vi "Serial connection test.vi"() -> ()   [LabVIEW 2024]
uses:
  664af4c5-80d0-43d0-860f-6e657b5a4ca0.vi
  <vilib>/regexp/Match Regular Expression.xnode
panel:
  out "error out":errorcluster
  out "find list":string[](array[string])
  in  "error in (no error)":errorcluster
  out "Device describtion":string[](array[string])
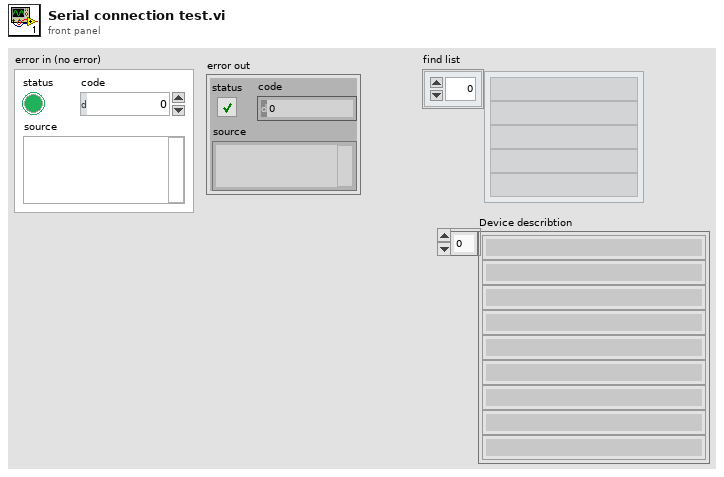
[diagram p1: front panel]
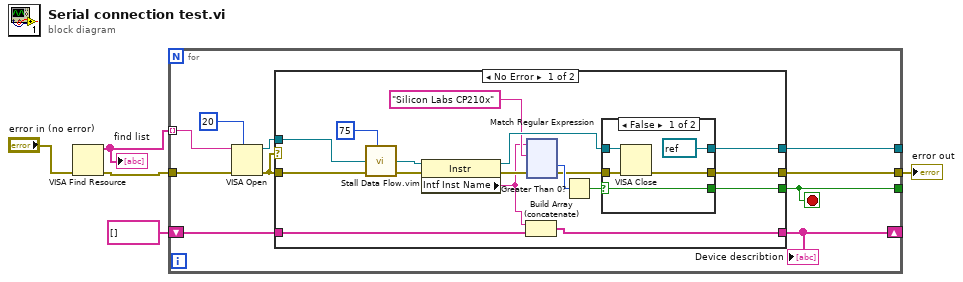
[diagram p0: block diagram]
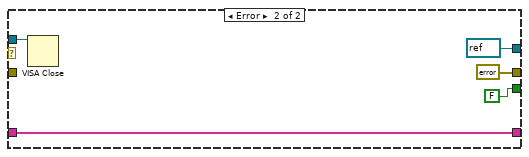
[diagram p3: hidden frame]
diagram:
  n1 = VISA Find Resource(8:"error in (no error)") -> (0:w4:errorcluster, 3:w5:string[])  [unwired: 2 in, 1 out]
  "find list" <- w5
  n2 = for {
    tunnel: w5 -> [w15] mode=indexing
    tunnel: w4 -> [w14]
    tunnel: [w11] -> w2
    tunnel: [w10] -> _
    tunnel: [w12] -> _
    shift-right: [w7] -> _
    shift-left: string[] [] -> [w6]
    stop <- w10 stop-if-true
    n3 = VISA Open(timeout (0)=u32 20 ("VISA Open timeout (0)"), error in (no error)=w14, VISA resource name=w15) -> (VISA resource name=w9:refnum<visa-resource-name>, error out=w13:errorcluster)  [unwired: 2 in]
    n4 = case shown="No Error" w13 {
      tunnel: w9 -> [w21 w159]
      tunnel: w13 -> [w31 _]
      tunnel: [w28 refnum<visa-resource-name> refnum ("Port")] -> w12
      tunnel: [w27 FALSE] -> w10
      tunnel: [w26 errorcluster {"status"=FALSE, "code"=0, "source"=""} ("error out")] -> w11
      tunnel: [w17 w157] -> w7
      tunnel: w6 -> [w16 w157]
      frame No Error {
        n5 = call "Stall Data Flow.vim"("value in"=w21, "milliseconds to wait"=u32 75) -> ("value out"=w20:refnum<visa-resource-name>)  [unwired: 1 out]
        n6 = property class="Instr"(reference=w20, error in=w31) -> (reference out=w29:refnum<visa-resource-name>, error out=w23:errorcluster, "Intf Inst Name"=w18:string)
        n7 = Build Array (concatenate)(w18, w16) -> (w17:string[])
        n8 = xnode "Match Regular Expression"("input string"=w18, "regular expression"="Silicon Labs CP210x", "error in"=w23) -> ("offset past match"=w24:i32, "error out"=w22:errorcluster)  [unwired: 3 in, 3 out]
        n9 = Greater Than 0?(x=w24) -> (x > 0?=w30:bool)
        n10 = case shown="False" w30 {
          selector: w30 -> [w153 w155]
          tunnel: w29 -> [w152 w156]
          tunnel: [refnum<visa-resource-name> refnum ("Port") w156] -> w28
          tunnel: [w153 w155] -> w27
          tunnel: w22 -> [w151 w154]
          tunnel: [w150 w154] -> w26
          frame False {
            n11 = VISA Close(VISA resource name=w152, error in (no error)=w151) -> (error out=w150:errorcluster)
          }
          frame True {
          }
        }
      }
      frame Error {
        n12 = VISA Close(VISA resource name=w159) -> ()  [unwired: 1 in, 1 out]
      }
    }
    "Device describtion" <- w7
  }
  "error out" <- w2
